vi "RenameDB.vi"(8 "error in (no error)":errorcluster, 10 "New File Name (with extension)":string, 11 "object in":refnum<class "TableLogger_CSV_Actor.lvclass">) -> (0 "error out":errorcluster, 3 "object out":refnum<class "TableLogger_CSV_Actor.lvclass">)   [LabVIEW 2014, in "TableLogger_CSV_Actor.lvlib" / "TableLogger_CSV_Actor.lvclass"]
uses:
  TableLogger_CSV_Actor.lvclass
  TableLogger_CSV_Actor.lvclass/TableLogger_CSV_Actor.ctl
  C/Program Files/National Instruments/LabVIEW 2018/user.lib/_OpenG.lib/file/file.llb/Strip Path - Traditional__ogtk.vi
  C/Program Files/National Instruments/LabVIEW 2018/user.lib/_OpenG.lib/file/file.llb/Build Path - Traditional__ogtk.vi
panel:
  # "Connector Pane"
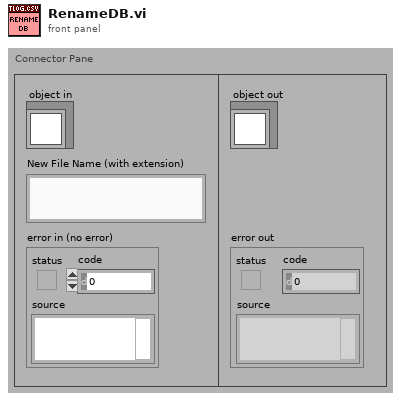
[diagram p1: front panel]
types:
  T1 = enum16{"open", "replace", "create", "open or create", "replace or create", "replace or create with confirmation"}
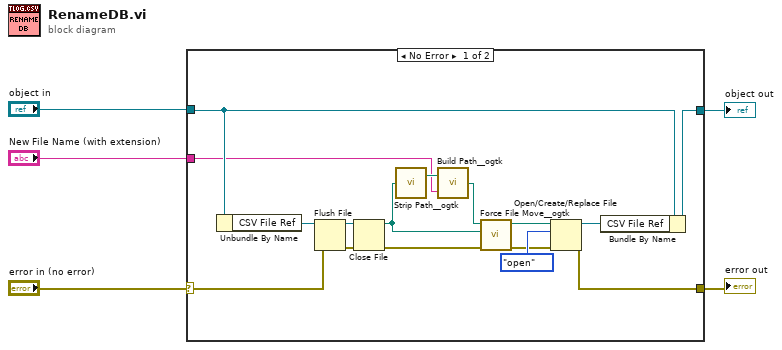
[diagram p0: block diagram]
diagram:
  n1 = case shown="No Error" "error in (no error)" {
    selector: "error in (no error)" -> [w10 w23]
    tunnel: [w9 w23] -> w4
    tunnel: [w20 w22] -> w2
    tunnel: "object in" -> [w21 w22]
    tunnel: "New File Name (with extension)" -> [w8 _]
    frame No Error {
      n2 = Unbundle By Name(w21) -> ("CSV File Ref"=w12:refnum<file>)
      n3 = Flush File(refnum=w12, error in=w10) -> (refnum out=w19:refnum<file>, error out=w16:errorcluster)
      n4 = Close File(refnum=w19, error in=w16) -> (path=w7:path, error out=w14:errorcluster)
      n5 = call-poly "Strip Path__ogtk.vi"("path"=w7) -> ("stripped path"=w15:path)  [unwired: 1 out]
      n6 = call-poly "Build Path__ogtk.vi"("name or relative path"=w8, "base path"=w15) -> ("appended path"=w6:path)
      n7 = call "Force File Move__ogtk.vi"("error in (no error)"=w14, "source"=w7, "target"=w6) -> ("error out"=w13:errorcluster, "target out"=w17:path)  [unwired: 3 in]
      n8 = Open/Create/Replace File(file path (use dialog)=w17, error in=w13, operation (0:open)=T1."open") -> (refnum out=w11:refnum<file>, error out=w9:errorcluster)  [unwired: 3 in, 1 out]
      n9 = Bundle By Name(cluster=w21, "CSV File Ref"=w11) -> (w20:refnum<class "TableLogger_CSV_Actor.lvclass">)
    }
    frame Error {
    }
  }
  "error out" <- w4
  "object out" <- w2
